vi "PH_gentec_Powermeter.set Sets 2 change Flag.vi"(0 "i ref in":refnum<vi>, 5 "error in":errorcluster) -> (14 "i ref out":refnum<vi>, 19 "error out":errorcluster)   [LabVIEW 2014, in "PH_gentec_Powermeter.lvlib"]
doc: "This VI indicates the wanted Settings at the GUI element."
uses:
  PH_gentec_Powermeter.lvlib
  PH_Powermeter_BaseClass/PH_Powermeter_BaseClass.State.ctl
  PH_Powermeter_BaseClass/PH_Powermeter_BaseClass.lvlib
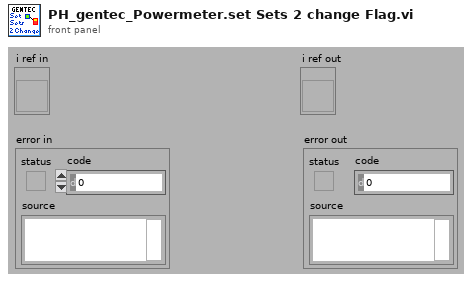
[diagram p1: front panel]
types:
  T1 = typedef "PH_Powermeter_BaseClass.lvlib/PH_Powermeter_BaseClass.i attribute.ctl" = cluster{"GUI References":T2, "Connection":T3, "Head Attributes":T5, "VISA resource":refnum<visa-resource-name>, "Energy":T6, "Service ID Energy":i32, "Wanted Settings":T7, "Current Settings":T7}
  T2 = typedef "PH_Powermeter_BaseClass.lvlib/PH_Powermeter_BaseClass.GUI Refs.ctl" = cluster{"Head Attributes":refnum<vi>, "Energy":refnum<vi>, "Connection":refnum<vi>, "VISA Resource":refnum<vi>, "Energy evolution":refnum<vi>, "Scaling Factor":refnum<vi>, "Range":refnum<vi>, "Wavelength":refnum<vi>, "Trigger Level":refnum<vi>, "Wanted Settings":refnum<vi>, "Current Settings":refnum<vi>}
  T3 = typedef "PH_Powermeter_BaseClass.lvlib/PH_Powermeter_BaseClass.Connection.ctl" = cluster{"failed checks":i8, "Timeout":bool, "Data read":string, "Failure":bool, "Error":bool, "State":T4}
  T4 = typedef "PH_Powermeter_BaseClass.lvlib/PH_Powermeter_BaseClass.State.ctl" = enum32{"off", "operating", "opened", "checked", "connected", "Sets to change", "running"}
  T5 = typedef "PH_Powermeter_BaseClass.lvlib/PH_Powermeter_BaseClass.Head Attributes.ctl" = cluster{"Instrument Type":string, "Head Version":string, "Head Name":string, "Serial Number":string, "Firmware":string, "Sensor Type":string, "MinimumRange":u32, "Maximum Range":u32, "Min Wavelength":i32, "Max Wavelength":i32}
  T6 = typedef "PH_Powermeter_BaseClass.lvlib/PH_Powermeter_BaseClass.Energy.ctl" = cluster{"current Value":dbl, "unscaled":dbl, "Scaling Factor":dbl}
  T7 = typedef "PH_Powermeter_BaseClass.lvlib/PH_gentec_BaseClass.Head Settings.ctl" = cluster{"Trigger Level":dbl, "Wavelength":u32, "Range":u32}
  T8 = typedef "PH_gentec_Powermeter.lvlib/PH_gentec_Powermeter.i attribute.ctl" = cluster{"GUI References":cluster{"delete":refnum<vi>, "start stop Statistics":refnum<vi>, "Statistic Data":refnum<vi>, "Configuration Values":refnum<vi>, "Set Zero":refnum<vi>, "Data Sampling Settings":refnum<vi>, "Wanted Sets":refnum<vi>, "Current Sets":refnum<vi>}, "Start Stop Statistics":bool, "Wanted Sets":T9, "Current Sets":T9}
  T9 = typedef "PH_gentec_Powermeter.lvlib/PH_gentec_Powermeter.Sets.ctl" = cluster{"Data Sampling Settings":T10, "Set Zero":bool}
  T10 = typedef "gentec-SOLO-PE - Driver.lvlib/gentec-SOLO-PE.Data Sampling Settings.ctl" = cluster{"Sample Rate":u32, "Sample Rate Unit":u32, "Sample Period":u32, "Sample Period Unit":u32, "Total Duration":u32, "Total Duration Unit":u32, "Time Stamp":u32}
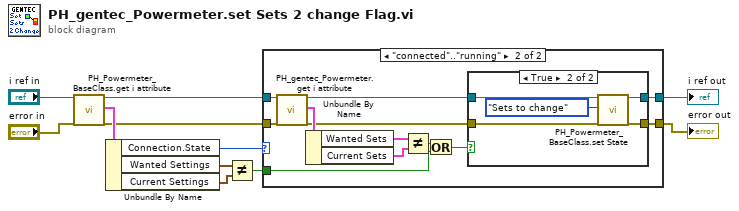
[diagram p0: block diagram]
diagram:
  n1 = call "PH_Powermeter_BaseClass.get i attribute.vi"("i ref in"="i ref in", "error in (no error)"="error in") -> ("i ref out"=w4:refnum<vi>, "i attribute"=w9:T1, "error out"=w3:errorcluster)  [unwired: 15 in]
  n2 = Unbundle By Name(w9) -> ("Connection.State"=w2:T4, "Wanted Settings"=w8:T7, "Current Settings"=w7:T7)
  n3 = Not Equal?(x=w8, y=w7) -> (x != y?=w1:bool)
  n4 = case shown="\"connected\"..\"running\"" w2 {
    tunnel: [w12 w22] -> w11
    tunnel: [w13 w21] -> w10
    tunnel: w4 -> [w13 w17]
    tunnel: w3 -> [w12 w16]
    tunnel: w1 -> [_ w14]
    frame Default {
    }
    frame "connected".."running" {
      n5 = call "PH_gentec_Powermeter.get i attribute.vi"("i ref in"=w17, "error in (no error)"=w16) -> ("i ref out"=w20:refnum<vi>, "i attribute"=w25:T8, "error out"=w19:errorcluster)  [unwired: 15 in]
      n6 = Unbundle By Name(w25) -> ("Wanted Sets"=w23:T9, "Current Sets"=w24:T9)
      n7 = Not Equal?(x=w23, y=w24) -> (x != y?=w18:bool)
      n8 = Or(x=w18, y=w14) -> (x .or. y?=w15:bool)
      n9 = case shown="True" w15 {
        tunnel: [w26 w32] -> w22
        tunnel: [w27 w31] -> w21
        tunnel: w20 -> [w27 w30]
        tunnel: w19 -> [w26 w29]
        frame False {
        }
        frame True {
          n10 = call "PH_Powermeter_BaseClass.set State.vi"("VI in"=w30, "State"=PH_Powermeter_BaseClass.State."Sets to change", "error in (no error)"=w29) -> ("VI out"=w31:refnum<vi>, "error out"=w32:errorcluster)  [unwired: 15 in]
        }
      }
    }
  }
  "error out" <- w11
  "i ref out" <- w10
